vi "Bisect Angle (scalar).vi"(7 "angle units":T1 items=["radian in, radian out", "radian in, degree out", "degree in, degree out", "degree in, radian out"], 9 "angle bisector range":T2=1 items=["none", "-180 to 180 (-pi to pi)", "0 to 360 (0 to 2pi)"], 10 "end angle":dbl, 11 "start angle":dbl) -> (0 "error":i32, 3 "angle bisector":dbl)   [LabVIEW 2017, in "NI_AAL_Angle.lvlib"]
doc: "Calculates the angle that bisects the start angle and the end angle into two equal parts.\n\nWire data to any of the angle inputs to determine the polymorphic instance to use or manually select the instance."
uses:
  <vilib>/Analysis/NI_AAL_Angle.lvlib
  <vilib>/Analysis/coordinate.llb/Angle Range (Degree).ctl
  <vilib>/Analysis/coordinate.llb/Angle Units.ctl
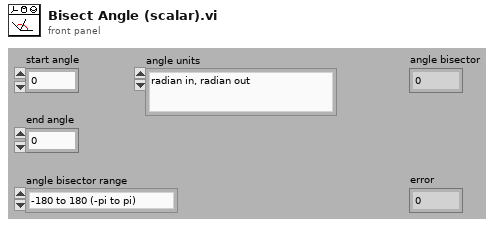
[diagram p1: front panel]
types:
  T1 = typedef "NI_AAL_Angle.lvlib/Angle Units.ctl" = i32
  T2 = typedef "NI_AAL_Angle.lvlib/Angle Range (Degree).ctl" = u16
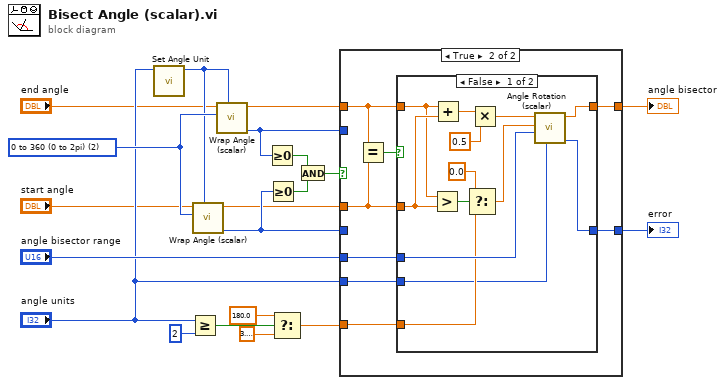
[diagram p0: block diagram]
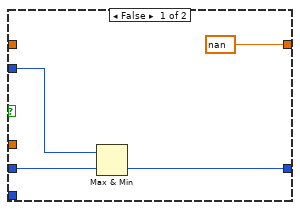
[diagram p2: hidden frame]
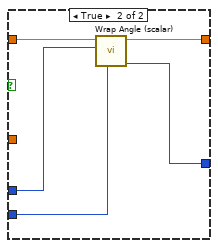
[diagram p3: hidden frame]
diagram:
  w20 = T2 2 items=["none", "-180 to 180 (-pi to pi)", "0 to 360 (0 to 2pi)"] ("angle range")
  n1 = call <vilib>:"Set Angle Unit.vi"("angle units in"="angle units") -> ("angle units out"=w3:T1)  [unwired: 10 in]
  n2 = Greater Or Equal?(x="angle units", y=2) -> (x >= y?=w8:bool)
  n3 = call <vilib>:"Wrap Angle (scalar).vi"("angle units"=w3, "angle range"=w20, "angle in"="start angle") -> ("error"=w15:i32, "angle out"=w11:dbl)  [unwired: 7 in]
  n4 = call <vilib>:"Wrap Angle (scalar).vi"("angle units"=w3, "angle range"=w20, "angle in"="end angle") -> ("error"=w16:i32, "angle out"=w12:dbl)  [unwired: 7 in]
  n5 = Greater Or Equal To 0?(x=w16) -> (x >= 0?=w19:bool)
  n6 = Greater Or Equal To 0?(x=w15) -> (x >= 0?=w18:bool)
  n7 = Select(t=180.0, s=w8, f=3.141592653589793) -> (s? t:f=w5:dbl)
  n8 = And(x=w19, y=w18) -> (x .and. y?=w17:bool)
  n9 = case shown="True" w17 {
    tunnel: w16 -> [w24 _]
    tunnel: w15 -> [w23 _]
    tunnel: [w22 w29] -> w14
    tunnel: [nan w30] -> w13
    tunnel: w12 -> [_ w31]
    tunnel: w11 -> [_ w26]
    tunnel: "angle bisector range" -> [_ w28]
    tunnel: "angle units" -> [_ w27]
    tunnel: w5 -> [_ w25]
    frame False {
      n10 = Max & Min(x=w24, y=w23) -> (min(x,y)=w22:i32)  [unwired: 1 out]
    }
    frame True {
      n11 = Equal?(x=w31, y=w26) -> (x = y?=w32:bool)
      n12 = case shown="False" w32 {
        tunnel: w31 -> [w38 w50]
        tunnel: [w41 w47] -> w30
        tunnel: [w40 w49] -> w29
        tunnel: w28 -> [w42 w48]
        tunnel: w27 -> [w33 w46]
        tunnel: w26 -> [w39 _]
        tunnel: w25 -> [w34 _]
        frame False {
          n13 = Greater?(x=w38, y=w39) -> (0:w37:bool)
          n14 = Add(x=w38, y=w39) -> (x+y=w45:dbl)
          n15 = Select(t=0.0, s=w37, f=w34) -> (s? t:f=w36:dbl)
          n16 = Multiply(x=w45, y=0.5) -> (x*y=w43:dbl)
          n17 = call <vilib>:"Angle Rotation (scalar).vi"("angle units"=w33, "rotated angle range"=w42, "counterclockwise rotation"=w36, "angle"=w43) -> ("error"=w40:i32, "rotated angle"=w41:dbl)  [unwired: 6 in]
        }
        frame True {
          n18 = call <vilib>:"Wrap Angle (scalar).vi"("angle units"=w46, "angle range"=w48, "angle in"=w50) -> ("error"=w49:i32, "angle out"=w47:dbl)  [unwired: 7 in]
        }
      }
    }
  }
  "angle bisector" <- w13
  "error" <- w14
